vi "Clear Peak Hold Value.vi"(8 "error in (no error)":errorcluster, 10 "Calculate Block (1: Calculate Block 1)":i32(ring)=1 items=["Calculate Block 1"=1, "Calculate Block 2"=2, "Calculate Block 3"=3, "Calculate Block 4"=4], 11 "VISA resource name":refnum<visa-resource-name>) -> (0 "error out":errorcluster, 3 "VISA resource name out":refnum<visa-resource-name>)   [LabVIEW 2014, in "Agilent U2000 Series.lvlib"]
doc: "Clears the peak hold value for a specified calculate block so that a new peak hold value can be set. \n\nNote:\nThis VI supports Agilent U2021/2XA and U2042XA/U2044XA/U2049XA models only."
uses:
  Agilent U2000 Series.lvlib
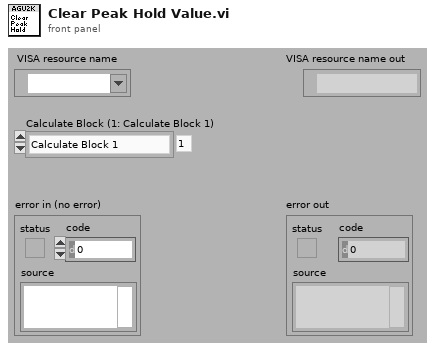
[diagram p1: front panel]
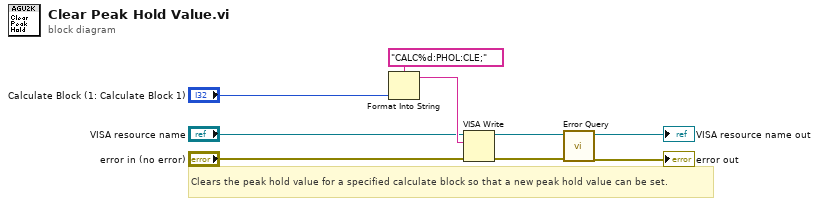
[diagram p0: block diagram]
diagram:
  # "Clears the peak hold value for a specified calculate block so that a new peak hold value can be set."
  n1 = Format Into String(format string="CALC%d:PHOL:CLE;", "Calculate Block (1: Calculate Block 1)") -> (resulting string=w7:string)  [unwired: 2 in, 1 out]
  n2 = VISA Write(VISA resource name="VISA resource name", write buffer=w7, error in (no error)="error in (no error)") -> (VISA resource name out=w4:refnum<visa-resource-name>, error out=w3:errorcluster)  [unwired: 1 out]
  n3 = call "Error Query.vi"("error in (no error)"=w3, "VISA resource name"=w4) -> ("error out"=→"error out":errorcluster, "VISA resource name out"=→"VISA resource name out":refnum<visa-resource-name>)  [unwired: 8 out]
